vi "Clear myVTOL.vi"(8 "Error In":errorcluster, 11 "task array in":refnum<k21>[](array[refnum])) -> (0 "Error Out":errorcluster)   [LabVIEW 2013]
doc: "Clears both DAQmx tasks created for the myQuake."
uses:
  <vilib>/DAQmx/write.llb/DAQmx Write (Analog DBL 1Chan 1Samp).vi
  <vilib>/DAQmx/miscellaneous.llb/DAQmx Fill In Error Info.vi
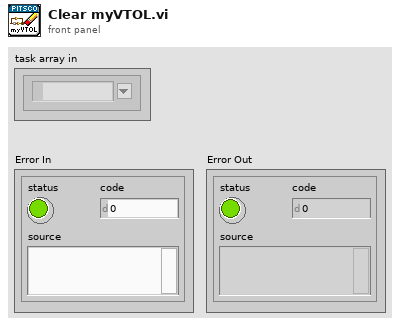
[diagram p1: front panel]
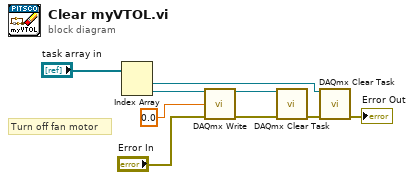
[diagram p0: block diagram]
diagram:
  # "Turn off fan motor"
  n1 = Index Array(array="task array in") -> (element #1=w4:refnum<k21>, element #2=w3:refnum<k21>)  [unwired: 2 in]
  n2 = call-poly <vilib>:"DAQmx Write.vi"("task/channels in"=w3, "data"=0.0, "error in"="Error In") -> ("task out"=w6:refnum<k21>, "error out"=w7:errorcluster)  [unwired: 10 in, 1 out]
  n3 = call <vilib>:"DAQmx Clear Task.vi"("task in"=w6, "error in"=w7) -> ("error out"=w9:errorcluster)  [unwired: 13 in]
  n4 = call <vilib>:"DAQmx Clear Task.vi"("task in"=w4, "error in"=w9) -> ("error out"=→"Error Out":errorcluster)  [unwired: 13 in]
